vi "Get Temperature Range.vi"(8 "error in (no error)":errorcluster, 10 "maxtemp":i32, 11 "mintemp":i32) -> (0 "error out":errorcluster, 1 "function return":u32, 2 "maxtemp out":i32, 3 "mintemp out":i32)   [LabVIEW 2014, in "atmcd32d.lvlib"]
doc: "unsigned int WINAPI GetTemperatureRange(int * mintemp, int * maxtemp);"
uses:
  atmcd32d.lvlib
  atmcd32d.dll
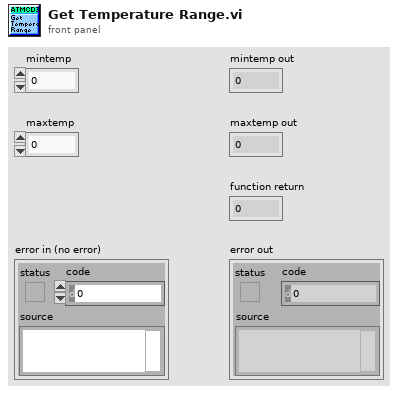
[diagram p1: front panel]
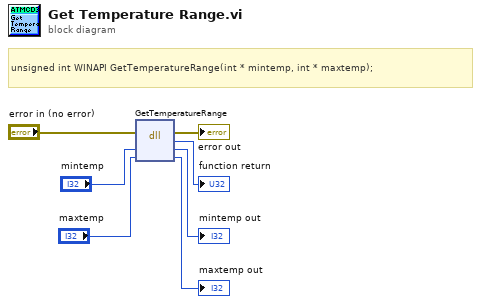
[diagram p0: block diagram]
diagram:
  # "unsigned int WINAPI GetTemperatureRange(int * mintemp, int * maxtemp);"
  n1 = dll-call lib="C:/Users/Bakir/Documents/Lambda2-Testing/lib/Andorlib/atmcd32d.*" fn="GetTemperatureRange"(error in="error in (no error)", "mintemp"="mintemp", "maxtemp"="maxtemp") -> (error out=→"error out":errorcluster, →"function return":u32, "mintemp"=→"mintemp out":i32, "maxtemp"=→"maxtemp out":i32)  [unwired: 2 in, 1 out]
